vi "dfd_Calculate Filter Scaling.vi"(5 "structure type":T2=enum."Lattice ARMA (basic sections)", 7 "scale type":T1=enum."Time Domain 1-Norm", 8 "gain":dbl, 9 "coef a/k":dbl[](array[numeric]) format="%.2f", 10 "coef b/v":dbl[](array[numeric]) format="%.2f", 11 "iterations":i32) -> (0 "scaled gain":dbl, 1 "scaled coefficients a/k":dbl[](array[numeric]) format="%.2f", 2 "scaled coefficients b/v":dbl[](array[numeric]) format="%.2f", 3 "input shift":i16)   [LabVIEW 2017, in "NI_DigFilter_FXP.lvlib"]
uses:
  <vilib>/addons/Digital Filter Design/NI_DigFilter_FXP.lvlib
  <vilib>/addons/Digital Filter Design/_Objects.llb/DFD Filter Structure Type Selector.ctl
  <vilib>/addons/Digital Filter Design/_Objects.llb/DFD Coef Norm Type.ctl
  <vilib>/addons/Digital Filter Design/NI_DigFilterLicensed.lvlib
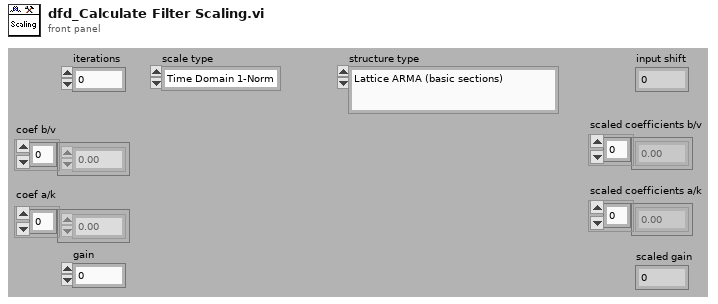
[diagram p1: front panel]
types:
  T1 = typedef "NI_DigFilterLicensed.lvlib/DFD Coef Norm Type.ctl" = enum16{"No Norm", "Time Domain 1-Norm", "Time Domain 2-Norm", "Time Domain Inf-Norm"}
  T2 = typedef "NI_DigFilterLicensed.lvlib/DFD Filter Structure Type Selector.ctl" = enum16{"Undefined", "FIR Direct Form", "FIR Direct Form Transposed", "FIR Symmetric", "FIR Antisymmetric", "IIR Direct Form I", "IIR Direct Form I Transposed", "IIR Direct Form II", "IIR Direct Form II Transposed", "IIR Cascaded Second Order Sections Form I", "IIR Cascaded Second Order Sections Form I Transposed", "IIR Cascaded Second Order Sections Form II", "IIR Cascaded Second Order Sections Form II Transposed", "Lattice Allpass (basic sections)", "Lattice Allpass (one multiplier sections)", "Lattice Allpass (normalized sections)", "Lattice AR (basic sections)", "Lattice AR (one multiplier sections)", "Lattice AR (normalized sections)", "Lattice MA (minimum phase)", "Lattice MA (maximum phase)", "Lattice ARMA (basic sections)", "Lattice ARMA (one multiplier sections)", "Lattice ARMA (normalized sections)"}
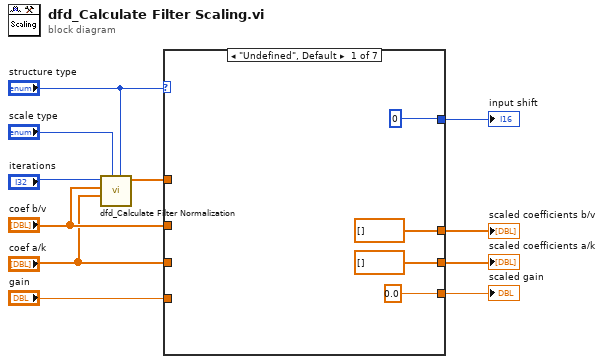
[diagram p0: block diagram]
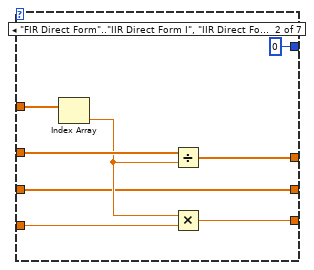
[diagram p2: hidden frame]
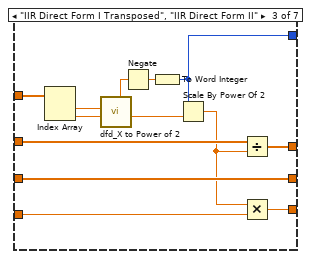
[diagram p3: hidden frame]
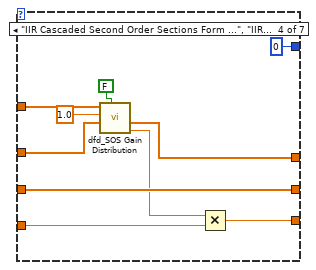
[diagram p4: hidden frame]
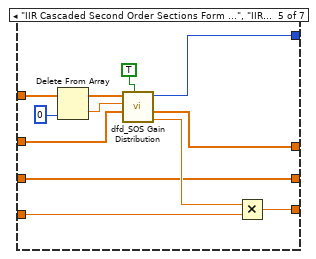
[diagram p5: hidden frame]
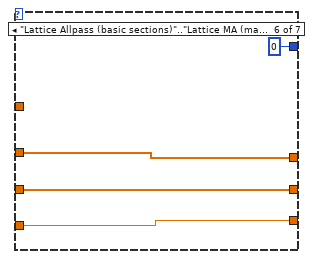
[diagram p6: hidden frame]
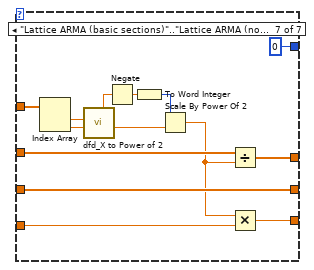
[diagram p7: hidden frame]
diagram:
  n1 = call <vilib>:"dfd_Calculate Filter Normalization.vi"("structure type"="structure type", "scale type"="scale type", "coefficients a/k"="coef a/k", "coefficients b/v"="coef b/v", "iterations"="iterations") -> ("norm"=w3:dbl[])  [unwired: 6 out]
  n2 = case shown="\"Undefined\", Default" "structure type" {
    tunnel: w3 -> [_ w22 w35 w43 w57 _ w73]
    tunnel: "coef a/k" -> [_ w16 w27 w39 w47 w61 w65]
    tunnel: "coef b/v" -> [_ w21 w29 w42 w52 w59 w67]
    tunnel: "gain" -> [_ w20 w25 w37 w50 w58 w63]
    tunnel: [dbl[] [] ("scaled coefficients a") w16 w27 w39 w47 w61 w65] -> w10
    tunnel: [dbl[] [] ("scaled coefficients b") w17 w28 w40 w51 w59 w66] -> w9
    tunnel: [0.0 ("scaled gain") w18 w24 w36 w49 w58 w62] -> w8
    tunnel: [i16 0 ("input shift") i16 0 ("input shift") w30 i16 0 ("input shift") w46 i16 0 ("input shift") i16 0 ("input shift")] -> w7
    frame "Undefined", Default {
    }
    frame "FIR Direct Form".."IIR Direct Form I", "IIR Direct Form II Transposed" {
      n3 = Index Array(array=w22) -> (element=w19:dbl)  [unwired: 1 in]
      n4 = Divide(x=w21, y=w19) -> (x/y=w17:dbl[])
      n5 = Multiply(x=w19, y=w20) -> (x*y=w18:dbl)
    }
    frame "IIR Direct Form I Transposed", "IIR Direct Form II" {
      n6 = Index Array(array=w35) -> (element #1=w34:dbl, element #2=w31:dbl)  [unwired: 2 in]
      n7 = call <vilib>:"dfd_X to Power of 2.vi"("x"=w34) -> ("n"=w32:dbl)  [unwired: 10 out]
      n8 = Negate(x=w32) -> (-x=w33:dbl)
      n9 = To Word Integer(number=w33) -> (16bit integer=w30:i16)
      n10 = Scale By Power Of 2(n=w30, x=w31) -> (x*2^n=w26:dbl)
      n11 = Divide(x=w29, y=w26) -> (x/y=w28:dbl[])
      n12 = Multiply(x=w26, y=w25) -> (x*y=w24:dbl)
    }
    frame "IIR Cascaded Second Order Sections Form I", "IIR Cascaded Second Order Sections Form II Transposed" {
      n13 = call <vilib>:"dfd_SOS Gain Distribution.vi"("power of 2 initial?"=FALSE, "coefficients b"=w42, "initial"=1.0, "norms"=w43) -> ("global gain"=w38:dbl, "scaled coefficients b"=w40:dbl[])  [unwired: 6 out]
      n14 = Multiply(x=w38, y=w37) -> (x*y=w36:dbl)
    }
    frame "IIR Cascaded Second Order Sections Form I Transposed", "IIR Cascaded Second Order Sections Form II" {
      n15 = Delete From Array(array=w57, index=0) -> (deleted portion=w53:dbl, array with subset deleted=w55:dbl[])  [unwired: 1 in]
      n16 = call <vilib>:"dfd_SOS Gain Distribution.vi"("power of 2 initial?"=TRUE, "coefficients b"=w52, "initial"=w53, "norms"=w55) -> ("global gain"=w48:dbl, "scaled coefficients b"=w51:dbl[], "input shift"=w46:i16)  [unwired: 5 out]
      n17 = Multiply(x=w48, y=w50) -> (x*y=w49:dbl)
    }
    frame "Lattice Allpass (basic sections)".."Lattice MA (maximum phase)" {
    }
    frame "Lattice ARMA (basic sections)".."Lattice ARMA (normalized sections)" {
      n18 = Index Array(array=w73) -> (element #1=w69:dbl, element #2=w68:dbl)  [unwired: 2 in]
      n19 = call <vilib>:"dfd_X to Power of 2.vi"("x"=w69) -> ("n"=w72:dbl)  [unwired: 10 out]
      n20 = Negate(x=w72) -> (-x=w71:dbl)
      n21 = To Word Integer(number=w71) -> (16bit integer=w70:i16)
      n22 = Scale By Power Of 2(n=w70, x=w68) -> (x*2^n=w64:dbl)
      n23 = Divide(x=w67, y=w64) -> (x/y=w66:dbl[])
      n24 = Multiply(x=w64, y=w63) -> (x*y=w62:dbl)
    }
  }
  "scaled coefficients a/k" <- w10
  "scaled coefficients b/v" <- w9
  "scaled gain" <- w8
  "input shift" <- w7
